vi "RTS Asyncrouns Read Solo.vi"(8 "error in (no error)":errorcluster, 11 "CSV File Location 8":path) -> (0 "error out":errorcluster, 3 "refnum out":refnum<file>)   [LabVIEW 2016]
panel:
  in  "Debug":bool
  out "Refnum out":refnum<k34>
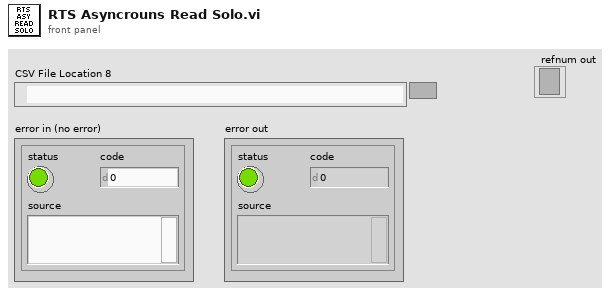
[diagram p1: front panel]
types:
  T1 = enum16{"open", "replace", "create", "open or create", "replace or create", "replace or create with confirmation"}
  T2 = enum16{"open", "open or create", "create or replace", "create", "open (read-only)"}
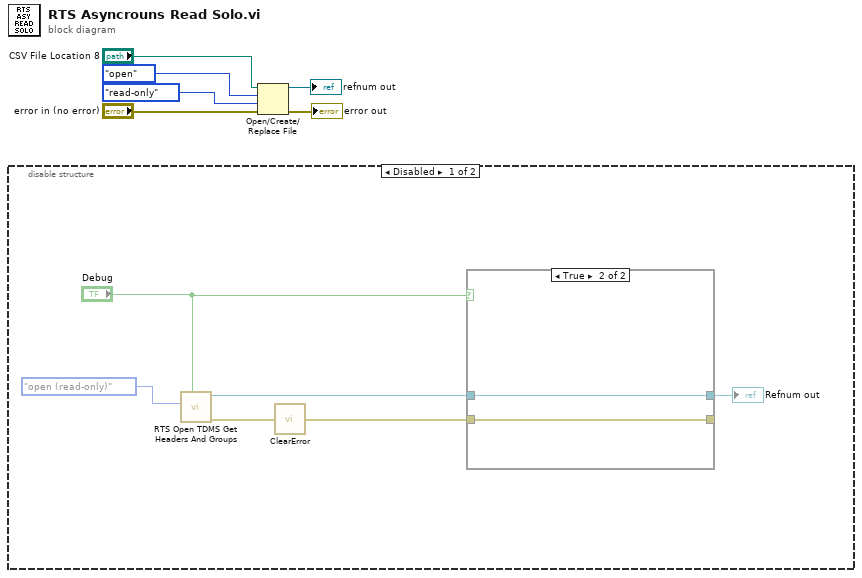
[diagram p0: block diagram]
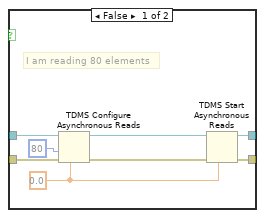
[diagram p2: hidden frame]
diagram:
  n1 = disable-structure shown="Disabled" {
    frame Disabled {
      n2 = call "RTS Open TDMS Get Headers And Groups.vi"("Debug"="Debug", "Operation"=T2."open (read-only)") -> ("Error Out"=w11:errorcluster, "Refnum out"=w12:refnum<k34>, "file path"=w9:path)  [unwired: 7 in]
      n3 = call <vilib>:"ClearError.vi"("error in (no error)"=w11) -> ("error out"=w13:errorcluster)
      n4 = case shown="True" "Debug" {
        tunnel: w13 -> [w19 w23]
        tunnel: [w18 w22] -> w8
        tunnel: w12 -> [w17 w22]
        tunnel: [w14 w23] -> _
        frame False {
          w20 = 0.0 ("i16")
          # "I am reading 80 elements"
          n5 = TDMS Configure Asynchronous Reads(6:w20, 8:w19, 9:u32 80 ("buffer size"), 11:w17) -> (0:w16:errorcluster, 3:w15:refnum<k34>)  [unwired: 2 in]
          n6 = TDMS Start Asynchronous Reads(6:w20, 8:w16, 11:w15) -> (0:w14:errorcluster, 3:w18:refnum<k34>)  [unwired: 1 in]
        }
        frame True {
        }
      }
      "Refnum out" <- w8
    }
    frame Enabled {
    }
  }
  n7 = Open/Create/Replace File(file path (use dialog)="CSV File Location 8", error in="error in (no error)", operation (0:open)=T1."open", access (0:read/write)=enum16{"read/write", "read-only", "write-only"}."read-only") -> (refnum out=→"refnum out":refnum<file>, error out=→"error out":errorcluster)  [unwired: 2 in, 1 out]
